vi "CustomDeviceUI.vi"() -> ()   [LabVIEW 2019, in "CustomDevice.lvclass"]
uses:
  CustomDevice.lvclass
  <vilib>/NI/Configuration Framework/Node/NodeRef.ctl
  <vilib>/NI/Configuration Framework/Node/NISE_CEF_Node.lvclass
  <vilib>/NI/AMC/Message Queue.ctl
  <vilib>/NI/AMC/Message.ctl
  <vilib>/NI/Tools/Keyed Array/KeyedArray.ctl
  <vilib>/NI/Configuration Framework/Node/UserEventRef.ctl
  <vilib>/NI/Configuration Framework/Controls/EventCluster.ctl
  C:/Program Files (x86)/National Instruments/LabVIEW 2019/vi.lib/NI/Configuration Framework/Node/NISE_CEF_Node.lvclass
  CustomDevice.lvclass/CustomDevice.ctl
  Read Main CD Properties.vi
  Write Main CD Properties.vi
  <vilib>/NI/AMC/Create Single Message.vi
  <vilib>/NI/AMC/Update Message Routing Info.vi
  <vilib>/NI/AMC/Send Message.vi
  <vilib>/NI/AMC/AMC.lvlib
  Configuration Tool.lvlib
  <vilib>/NI/Tools/Keyed Array/Tools_KeyedArray.lvlib
  <vilib>/NI/Configuration Framework/NISE_CEF_TreeControl.lvlib
panel:
  in  "Main UI Tab":enum32{"Custom Device"}(tab)
  in  "Help":bool
  in  "Custom Device Name":string
  in  "Main Page GUID":string
  in  "Custom Device Type":T1(ring)
  in  "Max Occurrences":i32
  in  "Version":string
  in  "user event":T2
  in  "main queue":T3
  in  "node ref":T4
  # "General Settings"
  # "Execution Settings"
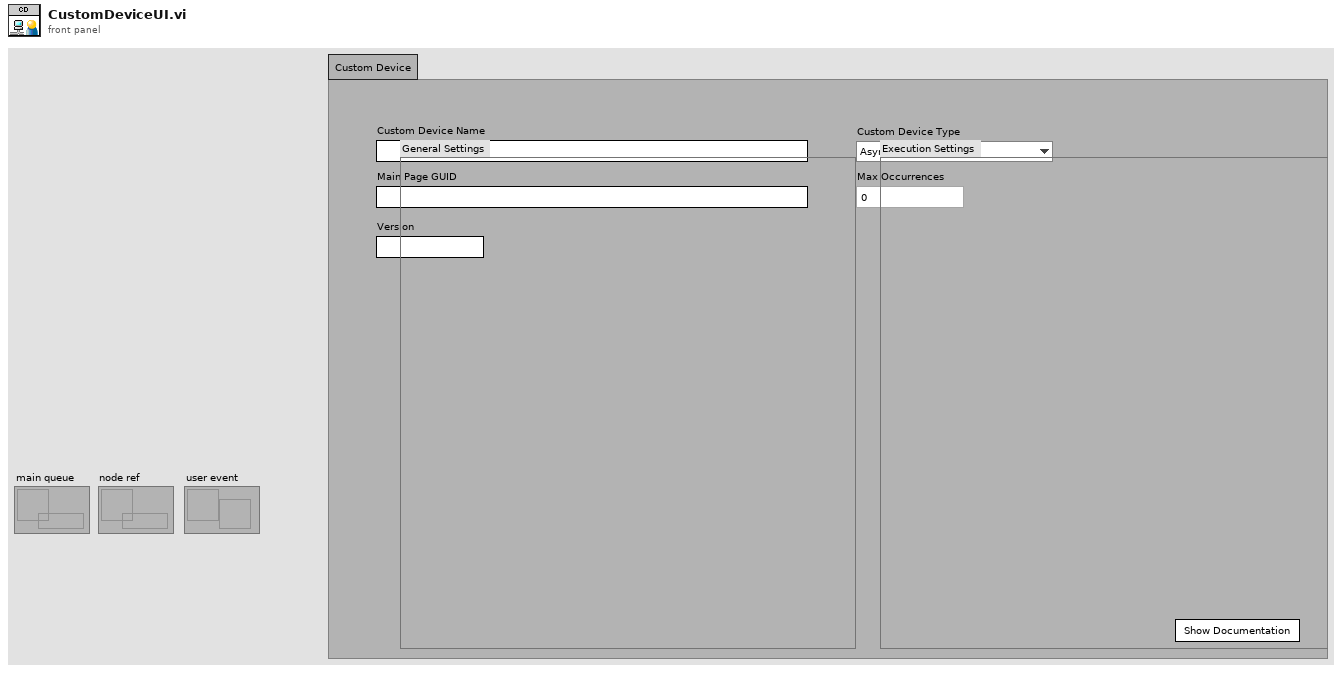
[diagram p1: front panel]
types:
  T1 = enum16{"Asynchronous", "Inline HW Interface", "Inline Model Interface", "Inline Timing and Sync", "Asynchronous Timing and Sync"}
  T2 = typedef "NISE_CEF_Node.lvclass/UserEventRef.ctl" = refnum<user-event>
  T3 = typedef "AMC.lvlib/Message Queue.ctl" = refnum<queue>
  T4 = typedef "NISE_CEF_Node.lvclass/NodeRef.ctl" = refnum<data-value>
  T5 = typedef "Main Custom Device Properties.ctl" = cluster{"CD Name":string, "Version":string, "Max Occurrences":i32, "Device Type":enum16{"Asynchronous", "Inline HW Interface", "Inline Model Interface", "Inline Timing and Sync", "Asynchronous Timing and Sync"}, "Main Page GUID":string}
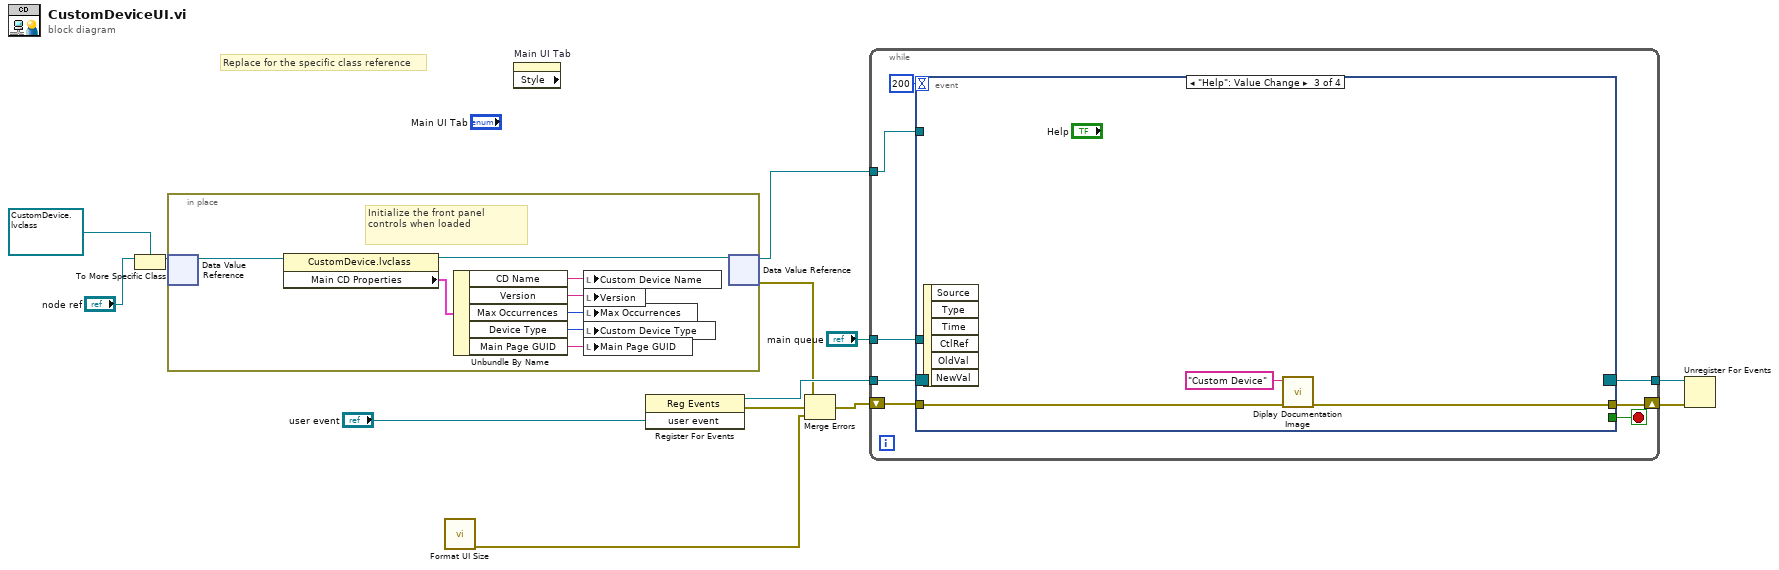
[diagram p0: block diagram]
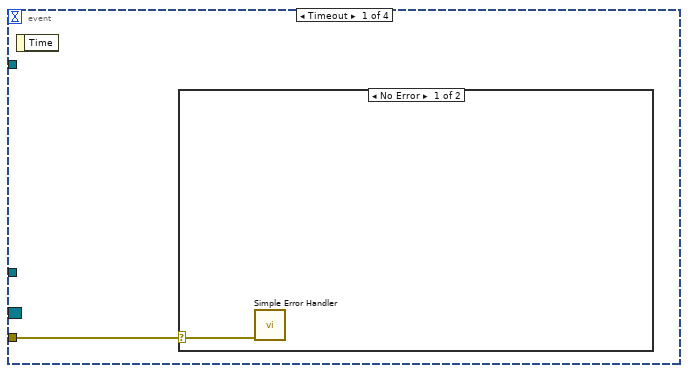
[diagram p2: hidden frame]
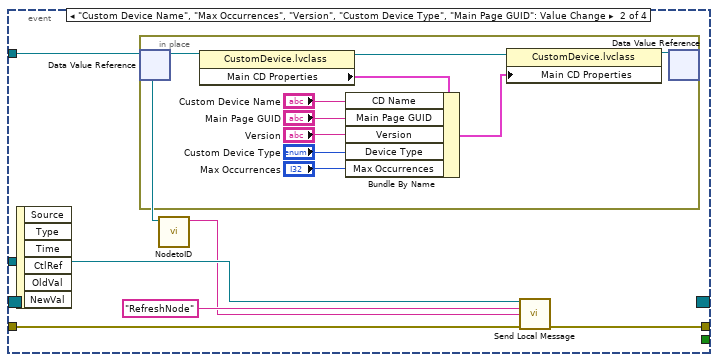
[diagram p4: hidden frame]
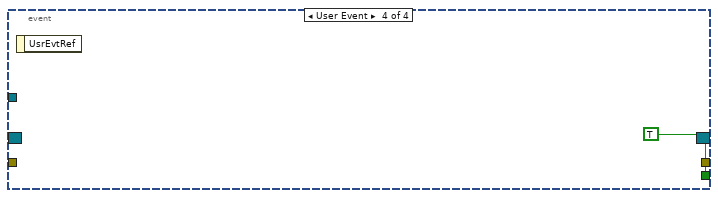
[diagram p5: hidden frame]
diagram:
  # "Replace for the specific class reference"
  n1 = To More Specific Class(target class=refnum<data-value> refnum ("data value reference"), reference="node ref") -> (specific class reference=w6:refnum<data-value>)  [unwired: 1 in, 1 out]
  n2 = in-place {
    # "Initialize the front panel controls when loaded"
    n3 = in-place-dvr #1(w6) -> (w21:refnum<class "CustomDevice.lvclass">)  [unwired: 1 out]
    n4 = property class="CustomDevice.lvclass"(reference=w21) -> (reference out=w20:refnum<class "CustomDevice.lvclass">, "Main CD Properties"=w19:T5)  [unwired: 1 in, 1 out]
    n5 = Unbundle By Name(w19) -> ("CD Name"=w18:string, "Version"=w17:string, "Max Occurrences"=w16:i32, "Device Type"=w15:T1, "Main Page GUID"=w14:string)
    n6 = local write "Custom Device Name"(w18) -> ()
    n7 = local write "Version"(w17) -> ()
    n8 = local write "Max Occurrences"(w16) -> ()
    n9 = local write "Custom Device Type"(w15) -> ()
    n10 = local write "Main Page GUID"(w14) -> ()
    n11 = in-place-dvr #1(w20) -> (w13:refnum<data-value>, w3:errorcluster)
  }
  n12 = call "Format UI Size.vi"() -> ("error out"=w1:errorcluster)  [unwired: 11 in]
  n13 = property on="Main UI Tab" class="TabCtl (strict)" props=["Style"]() -> ()  [unwired: 2 in, 3 out]
  n14 = register-events("user event") -> (reference out=w10:refnum<event-registration>, error out=w4:errorcluster)  [unwired: 2 in]
  n15 = Merge Errors(w3, w4, w1) -> (w2:errorcluster)
  n16 = while {
    tunnel: w13 -> [w29]
    tunnel: "main queue" -> [w28]
    tunnel: w10 -> [w26]
    tunnel: [w25] -> w9
    shift-right: [w23] -> w8
    shift-left: w2 -> [w22]
    stop <- w24 stop-if-true
    n17 = event shown="[2] \"Help\": Value Change" {
      selector: w26 -> [_ _ _ _]
      dyn-events: [_ _ _ _] -> w25
      timeout: 200 -> [_ _ _ _]
      tunnel: w29 -> [_ w35 _ _]
      tunnel: w28 -> [_ w36 _ _]
      tunnel: [_ _ _ TRUE] -> w24
      tunnel: [_ w33 w48 _] -> w23
      tunnel: w22 -> [w30 w32 w49 _]
      event Timeout {
        n18 = event-data() -> ()  [unwired: 1 in, 1 out]
        n19 = case shown="No Error" w30 {
          selector: w30 -> [w31 _]
          frame No Error {
            n20 = call <vilib>:"Simple Error Handler.vi"("error in (no error)"=w31) -> ()  [unwired: 4 in, 5 out]
          }
          frame Error {
          }
        }
      }
      event "Custom Device Name", "Max Occurrences", "Version", "Custom Device Type", "Main Page GUID": Value Change {
        n21 = event-data() -> ()  [unwired: 1 in, 6 out]
        n22 = in-place {
          n23 = in-place-dvr #2(w35) -> (w46:refnum<class "CustomDevice.lvclass">)  [unwired: 1 out]
          n24 = property class="CustomDevice.lvclass"(reference=w46) -> (reference out=w45:refnum<class "CustomDevice.lvclass">, "Main CD Properties"=w44:T5)  [unwired: 1 in, 1 out]
          n25 = Bundle By Name(cluster=w44, "CD Name"="Custom Device Name", "Main Page GUID"="Main Page GUID", "Version"="Version", "Device Type"="Custom Device Type", "Max Occurrences"="Max Occurrences") -> (w43:T5)
          n26 = property class="CustomDevice.lvclass"(reference=w45, "Main CD Properties"=w43) -> (reference out=w47:refnum<class "CustomDevice.lvclass">)  [unwired: 1 in, 1 out]
          n27 = in-place-dvr #2(w47) -> ()  [unwired: 2 out]
        }
        n28 = call <vilib>:"NodetoID.vi"("node ref"=w35) -> ("ID"=w34:string)  [unwired: 9 in, 1 out]
        n29 = call <vilib>:"Send Local Message.vi"("message queue in"=w36, "message name"="RefreshNode" ("Message Name"), "message value"=w34, "error in"=w32) -> ("error out"=w33:errorcluster)  [unwired: 9 in, 2 out]
      }
      event "Help": Value Change {
        n30 = event-data() -> ()  [unwired: 1 in, 6 out]
        n31 = call "Diplay Documentation Image.vi"("error in (no error)"=w49, "Image Name"="Custom Device") -> ("error out"=w48:errorcluster)  [unwired: 9 in]
      }
      event User Event {
        n32 = event-data() -> ()  [unwired: 1 in, 1 out]
      }
    }
  }
  n33 = Unregister For Events(event registration refnum=w9, error in=w8) -> ()  [unwired: 1 out]
